vi "Create Part Sample.vi"(8 "error in (no error)":errorcluster, 10 "Draw Style:Mode":T1(ring)=enum."Wireframe", 11 "Model":T2=enum."Utah Teapot") -> (0 "error out":errorcluster, 3 "XRay Part Sample out":refnum<class "XRay Part Sample.lvclass">)   [LabVIEW 2026, in "XRay Part Sample.lvclass"]
uses:
  XRay Part Sample.lvclass
  3D utilities/3DS Models.ctl
  XRay Part Sample.lvclass/XRay Part Sample.ctl
  <vilib>/picture/3D Picture Control/Object/Create Object (name).vi
  <vilib>/picture/3D Picture Control/Object/Add Object (no reference).vi
  <vilib>/picture/3D Picture Control/NI_3D Picture Control.lvlib
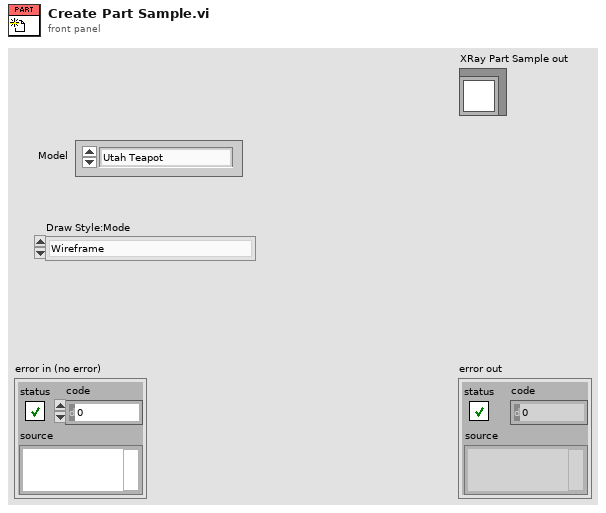
[diagram p1: front panel]
types:
  T1 = enum16{"Inherit Value", "Points", "Wireframe", "Polygons"}
  T2 = typedef "3DS Models.ctl" = enum16{"ASTM E2597 Step Wedge", "NI Bottle", "Utah Teapot", "Utah Teapot (Low Res)", "My Cube", "Tree", "Tree 2", "FreeCAD Sample", "Schenkel", "Bunny", "Corona Virus", "Corona Virus (Low Res)", "Offset"}
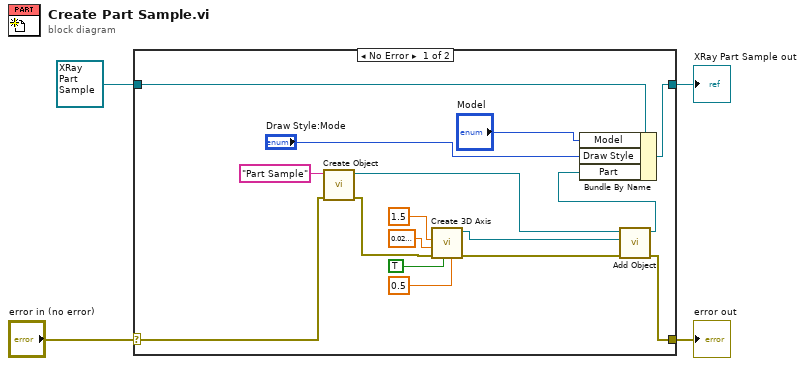
[diagram p0: block diagram]
diagram:
  n1 = case shown="No Error" "error in (no error)" {
    selector: "error in (no error)" -> [w17 w21]
    tunnel: [w7 w21] -> w3
    tunnel: [w19 w22] -> w2
    tunnel: refnum<class "XRay Part Sample.lvclass"> refnum ("XRay Part Sample in") -> [w20 w22]
    frame No Error {
      n2 = call-poly <vilib>:"Create Object.vi"("error in (no error)"=w17, "Name"="Part Sample") -> ("error out"=w8:errorcluster, "Scene:New Object"=w12:refnum<vi>)  [unwired: 8 in]
      n3 = call <vilib>:"Create 3D Axis.vi"("Character Size"=sgl 0.5, "Axis label?"=TRUE, "error in (no error)"=w8, "Radius"=sgl 0.03, "Length"=sgl 1.5 ("Height")) -> ("error out"=w9:errorcluster, "New Object Refnum"=w10:refnum<vi>)  [unwired: 5 in]
      n4 = call-poly <vilib>:"Add Object.vi"("error in (no error)"=w9, "New Object In"=w10, "Scene Object In"=w12) -> ("error out"=w7:errorcluster, "Scene Object Out"=w11:refnum<vi>)  [unwired: 7 in]
      n5 = Bundle By Name(cluster=w20, "Model"="Model", "Draw Style"="Draw Style:Mode", "Part"=w11) -> (w19:refnum<class "XRay Part Sample.lvclass">)
    }
    frame Error {
    }
  }
  "error out" <- w3
  "XRay Part Sample out" <- w2
